vi "Actor Example Callback.vi"(8 "error in (no error)":errorcluster, 9 "Scope":variant, 11 "Value":variant) -> (0 "error out":errorcluster)   [LabVIEW 2017, in "Actor Example.lvlib"]
uses:
  Actor Example.lvlib
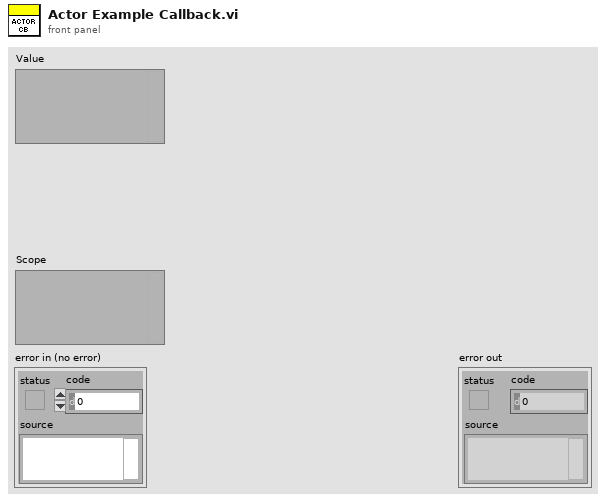
[diagram p1: front panel]
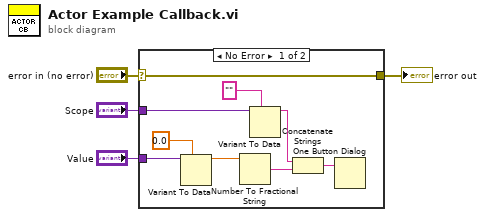
[diagram p0: block diagram]
diagram:
  n1 = case shown="No Error" "error in (no error)" {
    selector: "error in (no error)" -> [w13 w14]
    tunnel: [w13 w14] -> w3
    tunnel: "Scope" -> [w11 _]
    tunnel: "Value" -> [w12 _]
    frame No Error {
      n2 = Variant To Data(type=0.0 ("Threshold"), Variant=w12) -> (data=w6:dbl)  [unwired: 1 in, 1 out]
      n3 = Number To Fractional String(number=w6) -> (F-format string=w5:string)  [unwired: 3 in]
      n4 = Variant To Data(type="", Variant=w11) -> (data=w9:string)  [unwired: 1 in, 1 out]
      n5 = Concatenate Strings(w9, w5) -> (w8:string)
      n6 = One Button Dialog(message=w8) -> ()  [unwired: 1 in, 1 out]
    }
    frame Error {
    }
  }
  "error out" <- w3
